vi "getMarriedWomanExpression.vi"() -> (3 "AndExpression":refnum<class "AndExpression.lvclass">)   [LabVIEW 2018, in "InterpreterPatternDemo.lvclass"]
uses:
  InterpreterPatternDemo.lvclass
  AndExpression Class/AndExpression.lvclass
  TerminalExpression Class/TerminalExpression.lvclass
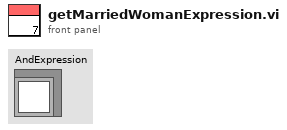
[diagram p1: front panel]
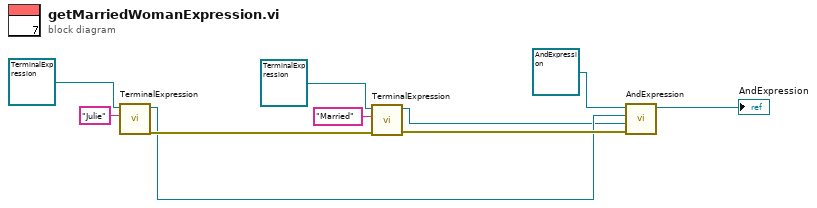
[diagram p0: block diagram]
diagram:
  n1 = call "TerminalExpression.vi"("data"="Julie", "TerminalExpression in"=refnum<class "TerminalExpression.lvclass"> refnum ("TerminalExpression.lvclass")) -> ("error out"=w6:errorcluster, "TerminalExpression out"=w4:refnum<class "TerminalExpression.lvclass">)  [unwired: 8 in]
  n2 = call "TerminalExpression.vi"("error in (no error)"=w6, "data"="Married", "TerminalExpression in"=refnum<class "TerminalExpression.lvclass"> refnum ("TerminalExpression.lvclass")) -> ("error out"=w5:errorcluster, "TerminalExpression out"=w3:refnum<class "TerminalExpression.lvclass">)  [unwired: 7 in]
  n3 = call "AndExpression.vi"("error in (no error)"=w5, "expr2"=w3, "expr1"=w4, "AndExpression in"=refnum<class "AndExpression.lvclass"> refnum ("AndExpression.lvclass")) -> ("AndExpression out"=→"AndExpression":refnum<class "AndExpression.lvclass">)  [unwired: 6 in, 1 out]
